vi "initialize.vi"(0 "HGF_Event":refnum<class "HGF_Event.lvclass">, 3 "initializationData":variant, 5 "error in (no error)":errorcluster, 7 "binaryString":string, 8 "I8 Array":i8[](array[numeric]), 9 "prependSize? (T)":bool, 11 "byteOrder (0:big-endian, network order)":T1(ring)) -> (14 "dup HGF_Event":refnum<class "HGF_Event.lvclass">, 17 "found?":bool, 19 "error out":errorcluster)   [LabVIEW 2014, in "HGF_BaseClasses.lvlib" / "HGF_Event.lvclass"]
doc: "This is a dynamic dispatch VI to be implemented by child classes to initialize their attributes.\n\n<B>Recommendation:</B> Use Variant for initialization data."
uses:
  HGF_Event.lvclass
  HGF_Base/HGF_Base.lvclass
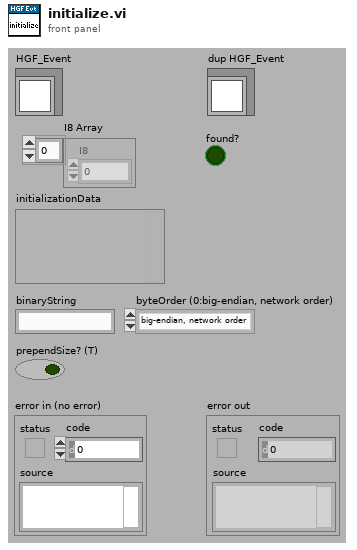
[diagram p1: front panel]
types:
  T1 = enum16{"big-endian, network order", "native, host order", "little-endian"}
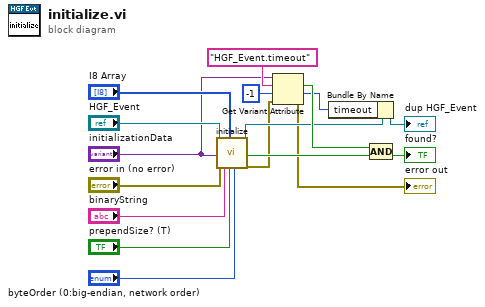
[diagram p0: block diagram]
diagram:
  n1 = call-parent "initialize.vi"("HGF_Base"="HGF_Event", "initializationData"="initializationData", "error in (no error)"="error in (no error)", "binaryString"="binaryString", "I8 Array"="I8 Array", "prependSize? (T)"="prependSize? (T)", "byteOrder (0:big-endian, network order)"="byteOrder (0:big-endian, network order)") -> ("dup HGF_Base"=w8:refnum<class "HGF_Event.lvclass">, "found?"=w10:bool, "error out"=w5:errorcluster)  [unwired: 1 in, 9 out]
  n2 = Get Variant Attribute(Variant="initializationData", name="HGF_Event.timeout", default value (empty Variant)=-1 ("timeout in ms (-1)"), error in=w5) -> (found=w11:bool, value=w7:i32, error out=→"error out":errorcluster)  [unwired: 1 out]
  n3 = Bundle By Name(cluster=w8, "timeout"=w7) -> (→"dup HGF_Event":refnum<class "HGF_Event.lvclass">)
  n4 = Compound Arithmetic op=AND(w11, w10) -> (→"found?":bool)
